vi "GEOM_MoveHeaders2.vi"   [LabVIEW 2016]
uses:
  GEOM_VAR_action.ctl
  GEOM_Gbls.vi
types:
  T1 = typedef "GEOM_VAR_action.ctl" = enum16{"read", "write"}
  T2 = typedef "GEOM_ReadModeHeader.ctl" = cluster{"readmode":string, "ME Headers":string[][][], "S Headers":string[][]}
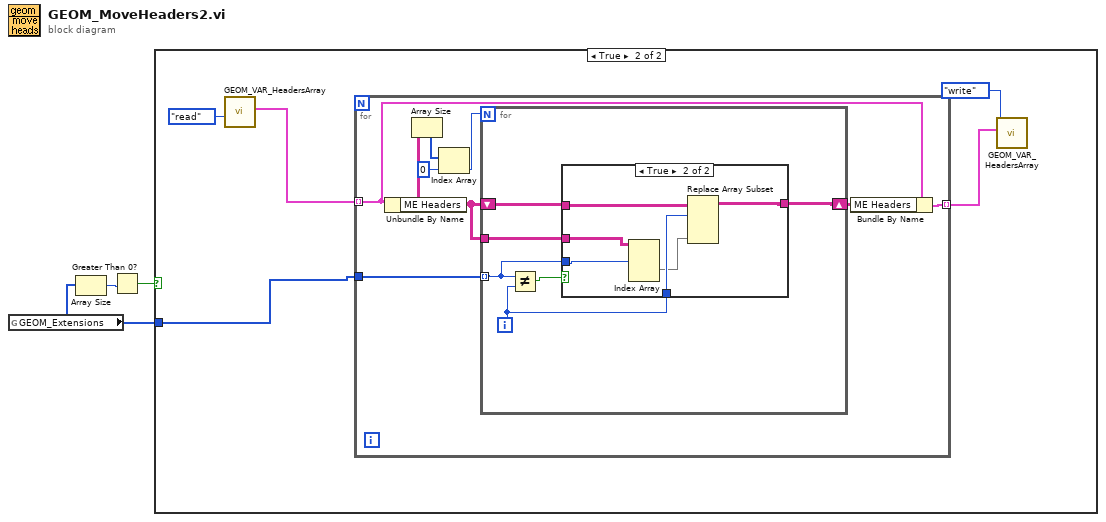
[diagram p0: block diagram]
diagram:
  n1 = global read "GEOM_Gbls.vi" "GEOM_Extensions"() -> (w3:i32[])
  n2 = Array Size(array=w3) -> (size(s)=w2:i32)
  n3 = Greater Than 0?(x=w2) -> (x > 0?=w1:bool)
  n4 = case shown="True" w1 {
    tunnel: w3 -> [_ w8]
    frame False {
    }
    frame True {
      n5 = call "GEOM_VAR_HeadersArray.vi"("Action"=GEOM_VAR_action."read") -> ("GEOM_HeadersArray out"=w5:T2[])  [unwired: 1 in, 9 out]
      n6 = for {
        tunnel: w8 -> [w16]
        tunnel: w5 -> [w14] mode=indexing
        tunnel: [w13] -> w7 mode=indexing
        n7 = Unbundle By Name(w14) -> ("ME Headers"=w12:string[][][])
        n8 = Array Size(array=w12) -> (size(s)=w11:i32[])
        n9 = Index Array(array=w11, index=0) -> (element=w9:i32)
        n10 = for {
          N: w9 -> [_]
          tunnel: w16 -> [w21] mode=indexing
          shift-right: [w17] -> w15
          shift-left: w12 -> [w19]
          tunnel: w12 -> [w18]
          i -> [w20]
          n11 = Not Equal?(x=w21, y=w20) -> (x != y?=w22:bool)
          n12 = case shown="True" w22 {
            tunnel: w19 -> [w23 w28]
            tunnel: [w23 w27] -> w17
            tunnel: w21 -> [_ w25]
            tunnel: w20 -> [_ w29]
            tunnel: w18 -> [_ w26]
            frame False {
            }
            frame True {
              n13 = Index Array(array=w26, index (dim 0)=w25) -> (element=w24:string[][])  [unwired: 2 in]
              n14 = Replace Array Subset(array=w28, new element=w24, index (dim 0)=w29) -> (w27:string[][][])  [unwired: 2 in]
            }
          }
        }
        n15 = Bundle By Name(cluster=w14, "ME Headers"=w15) -> (w13:T2)
      }
      n16 = call "GEOM_VAR_HeadersArray.vi"("Action"=GEOM_VAR_action."write", "GEOM_HeadersArray"=w7) -> ()  [unwired: 10 out]
    }
  }
